vi "Set Sample Rate.vi"(8 "error in (no error)":errorcluster, 10 "Sample Rate":u32 format="%#.12p", 11 "RTL-SDR in":refnum<class "Session.lvclass">) -> (0 "error out":errorcluster, 3 "RTL-SDR out":refnum<class "Session.lvclass">)   [LabVIEW 2020, in "RTL-SDR.lvlib" / "Session.lvclass"]
uses:
  Session.lvclass
  Session.lvclass/Session.ctl
  lib/librtlsdr.dll
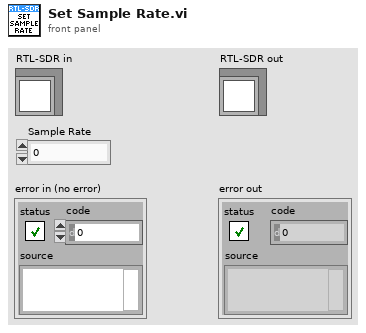
[diagram p1: front panel]
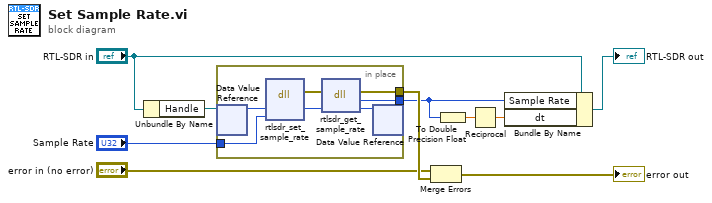
[diagram p0: block diagram]
diagram:
  n1 = Unbundle By Name("RTL-SDR in") -> ("Handle"=w1:refnum<data-value>)
  n2 = in-place {
    in-place-border: [w17] -> w10
    in-place-border: "Sample Rate" -> [w16]
    in-place-border: [w13] -> w4
    n3 = in-place-dvr #1(w1) -> (w11:u64)  [unwired: 1 out]
    n4 = dll-call lib="C:/dev/IlluminatedG/lv-rtl-sdr/lib/librtlsdr.dll" fn="rtlsdr_set_sample_rate"("dev"=w11, "rate"=w16) -> (error out=w15:errorcluster, "dev"=w14:u64)  [unwired: 5 in, 1 out]
    n5 = dll-call lib="C:/dev/IlluminatedG/lv-rtl-sdr/lib/librtlsdr.dll" fn="rtlsdr_get_sample_rate"(error in=w15, "dev"=w14) -> (error out=w17:errorcluster, "return type"=w13:u32, "dev"=w12:u64)  [unwired: 2 in, 1 out]
    n6 = in-place-dvr #1(w12) -> ()  [unwired: 2 out]
  }
  n7 = Merge Errors("error in (no error)", w10) -> (→"error out":errorcluster)
  n8 = To Double Precision Float(number=w4) -> (double precision float=w2:dbl)
  n9 = Reciprocal(x=w2) -> (1/x=w3:dbl)
  n10 = Bundle By Name(cluster="RTL-SDR in", "Sample Rate"=w4, "dt"=w3) -> (→"RTL-SDR out":refnum<class "Session.lvclass">)
